vi "LVClass_HasoEngine Get Preferences Multi Aperture.vi"(0 "HasoEngine in":refnum<class "HasoEngine.lvclass">, 11 "error in (no error)":errorcluster) -> (4 "HasoEngine out":refnum<class "HasoEngine.lvclass">, 6 "Start sub-aperture Array":T1[](array[typedef]), 8 "Pupil average":dbl=0.5 min=0.0 max=1.0, 10 "AutoStartSub-aperture":bool, 15 "error out":errorcluster)   [LabVIEW 2020, in "HasoEngine.lvclass"]
doc: "HasoSlopes computation preferences getter.\n\n--------------------------------------------------------------------------------\n\n<B>HasoEngineIn </B> : HasoEngine object.\n<B>HasoEngineOut </B> : HasoEngine object.\n<B>start_subpupil Array </B> : Array of coordinates of sub-pupil use to compute in multi aperture (index coordinates relative to the top-left corner of the pupil).\n<B>denoising_strength </B> : Sensitivity of spot detection on summed images (between 0 and 1).\n<B>auto_start </B> : Activation of the auto start subpupil detection in case specified start subpupil is not found\n<B>ErrorIn </B> : Error\n<B>ErrorOut </B> : Error\n\n--------------------------------------------------------------------------------"
uses:
  HasoEngine.lvclass
  Controls/Point2D.ctl
  HasoEngine.lvclass/HasoEngine.ctl
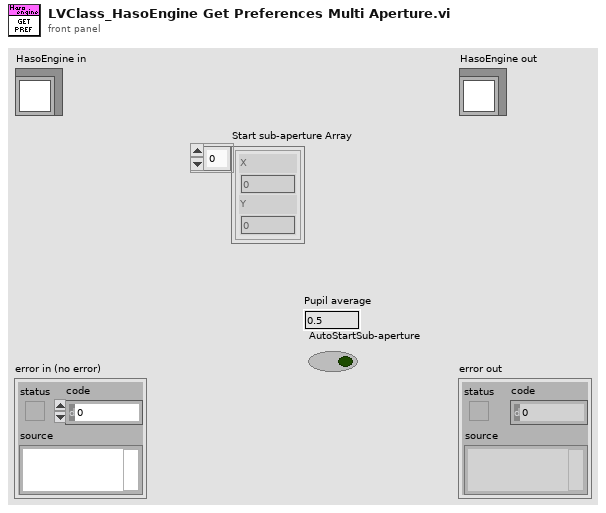
[diagram p1: front panel]
types:
  T1 = typedef "Point2D.ctl" = cluster{"X":u32, "Y":u32}
  T2 = typedef "ClassID.ctl" = i64
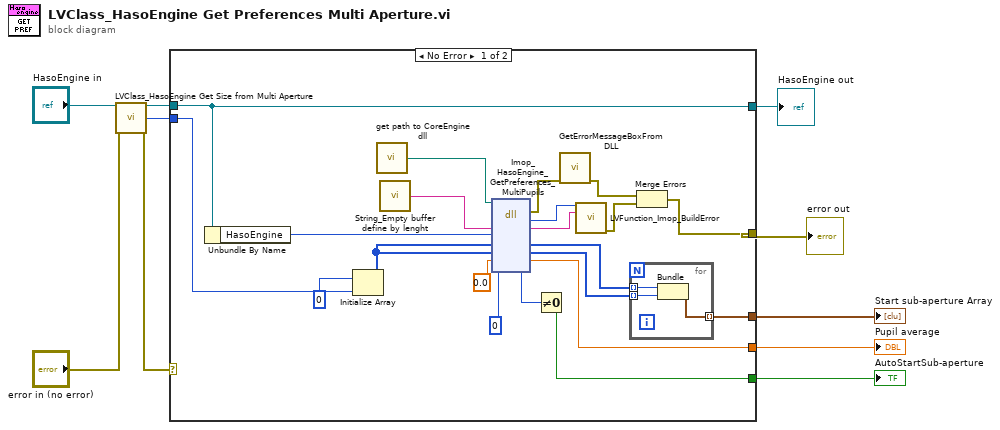
[diagram p0: block diagram]
diagram:
  n1 = call "LVClass_HasoEngine Get Size from Multi Aperture.vi"("HasoEngine in"="HasoEngine in", "error in (no error)"="error in (no error)") -> ("HasoEngine out"=w2:refnum<class "HasoEngine.lvclass">, "Size"=w1:i32, "error out"=w4:errorcluster)  [unwired: 11 in]
  n2 = case shown="No Error" w4 {
    selector: w4 -> [_ w35]
    tunnel: w2 -> [w25 w36]
    tunnel: [w25 w36] -> w9
    tunnel: [w21 w35] -> w10
    tunnel: [w18 _] -> w8
    tunnel: [w17 _] -> w7
    tunnel: [w11 _] -> w6
    tunnel: w1 -> [w16 _]
    frame No Error {
      n3 = Unbundle By Name(w25) -> ("HasoEngine"=w24:T2)
      n4 = Initialize Array(u32 0 ("X"), w16) -> (w14:u32[])
      n5 = call "get path to CoreEngine dll.vi"() -> ("path to wavekit library"=w28:path)  [unwired: 14 in, 1 out]
      n6 = call "String_Empty buffer define by lenght.vi"() -> ("Empty buffer"=w29:string)  [unwired: 1 in]
      n7 = dll-call lib="D:/2_trunk/Soft_haso/ImOpCoreEngine4_LV2011/DLLs/ImopEngine4_vc100.dll" fn="Imop_HasoEngine_GetPreferences_MultiPupils"(path in=w28, "message"=w29, "objet"=w24, "ArrayOfStartSubPupil_X"=w14, "ArrayOfStartSubPupil_Y"=w14, "pupil_average"=sgl 0.0, "AutoStartSub-aperture"=u8 0) -> (error out=w27:errorcluster, "return type"=w30:i32, "message"=w31:string, "ArrayOfStartSubPupil_X"=w12:u32[], "ArrayOfStartSubPupil_Y"=w13:u32[], "pupil_average"=w17:sgl, "AutoStartSub-aperture"=w20:u8)  [unwired: 3 in, 1 out]
      n8 = Not Equal To 0?(x=w20) -> (x != 0?=w18:bool)
      n9 = call "GetErrorMessageBoxFromDLL.vi"("error IN"=w27) -> ("error OUT"=w23:errorcluster)  [unwired: 10 in]
      n10 = call "LVFunction_Imop_BuildError.vi"("code"=w30, "String to Prepend to source (\"\")"=w31) -> ("error out"=w22:errorcluster)  [unwired: 13 in]
      n11 = for {
        tunnel: w12 -> [w34] mode=indexing
        tunnel: w13 -> [w33] mode=indexing
        tunnel: [w32] -> w11 mode=indexing
        n12 = Bundle(w34, w33) -> (w32:cluster{u32, u32})  [unwired: 1 in]
      }
      n13 = Merge Errors(w23, w22) -> (w21:errorcluster)
    }
    frame Error {
    }
  }
  "error out" <- w10
  "HasoEngine out" <- w9
  "Start sub-aperture Array" <- w6
  "Pupil average" <- w7
  "AutoStartSub-aperture" <- w8
